vi "标样核查配置.vi"() -> (2 "确认输出":bool)   [LabVIEW 2022 SP3, in "斯坦道多参数.lvlib"]
panel:
  in  "余氯标样值":dbl caption="余氯"
  in  "余氯启用":bool
  in  "水中油标样值":dbl caption="水中油"
  in  "水中油启用":bool
  in  "悬浮物标样值":dbl caption="悬浮物"
  in  "悬浮物启用":bool
  in  "氨氮标样值":dbl caption="氨氮"
  in  "COD标样值":dbl caption="COD"
  in  "氨氮启用":bool
  in  "COD启用":bool
  in  "氯化物标样值":dbl caption="氯化物"
  in  "氯化物启用":bool
  in  "ORP标样值":dbl caption="ORP"
  in  "ORP启用":bool
  in  "藻密度标样值":dbl caption="藻密度"
  in  "叶绿素a标样值":dbl caption="叶绿素a"
  in  "藻密度启用":bool
  in  "叶绿素a启用":bool
  in  "保存组数":dbl=1.0
  in  "浊度启用":bool
  in  "电导率启用":bool
  in  "溶解氧启用":bool
  in  "pH启用":bool
  in  "浊度标样值":dbl caption="浊度"
  in  "电导率标样值":dbl caption="电导率"
  in  "溶解氧标样值":dbl caption="溶解氧"
  in  "pH标样值":dbl caption="pH"
  in  "取消":bool
  in  "确定":bool
  in  "数据保存间隔":dbl=1.0
  # "请输入数据保存间隔"
  # "保存组数"
  # "min"
  # "组"
  # "请选择启动项"
  # "请输入各参数标样值"
  # "mg/L"
  # "μS/cm"
  # "NTU"
  # "μg/L"
  # "cells/mL"
  # "mg/L"
  # "mg/L"
  # "mg/L"
  # "mg/L"
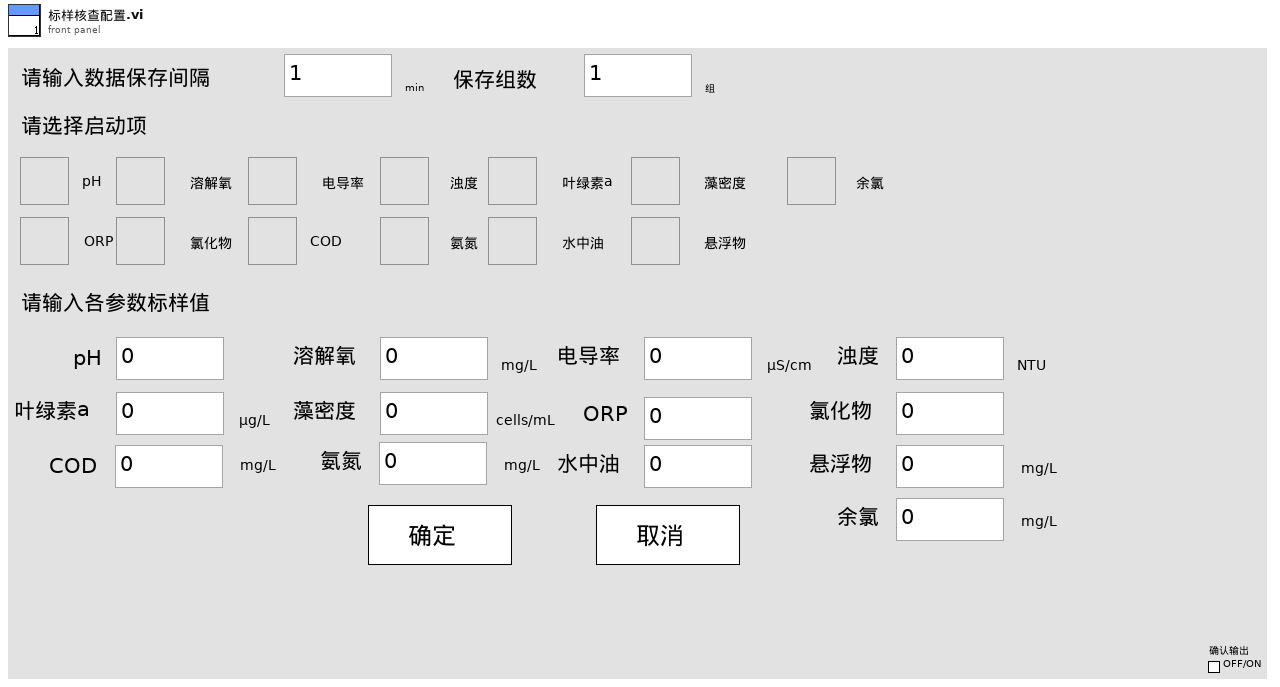
[diagram p1: front panel]
types:
  T1 = cluster{"数据保存间隔":dbl, "保存组数":dbl, "水温标样值":dbl, "pH标样值":dbl, "溶解氧标样值":dbl, "电导率标样值":dbl, "浊度标样值":dbl, "悬浮物标样值":dbl, "叶绿素a标样值":dbl, "藻密度标样值":dbl, "ORP标样值":dbl, "氯化物标样值":dbl, "COD标样值":dbl, "氨氮标样值":dbl, "水中油标样值":dbl, "余氯标样值":dbl, "pH启用":bool, "溶解氧启用":bool, "电导率启用":bool, "浊度启用":bool, "悬浮物启用":bool, "叶绿素a启用":bool, "藻密度启用":bool, "ORP启用":bool, "氯化物启用":bool, "COD启用":bool, "氨氮启用":bool, "水中油启用":bool, "余氯启用":bool}
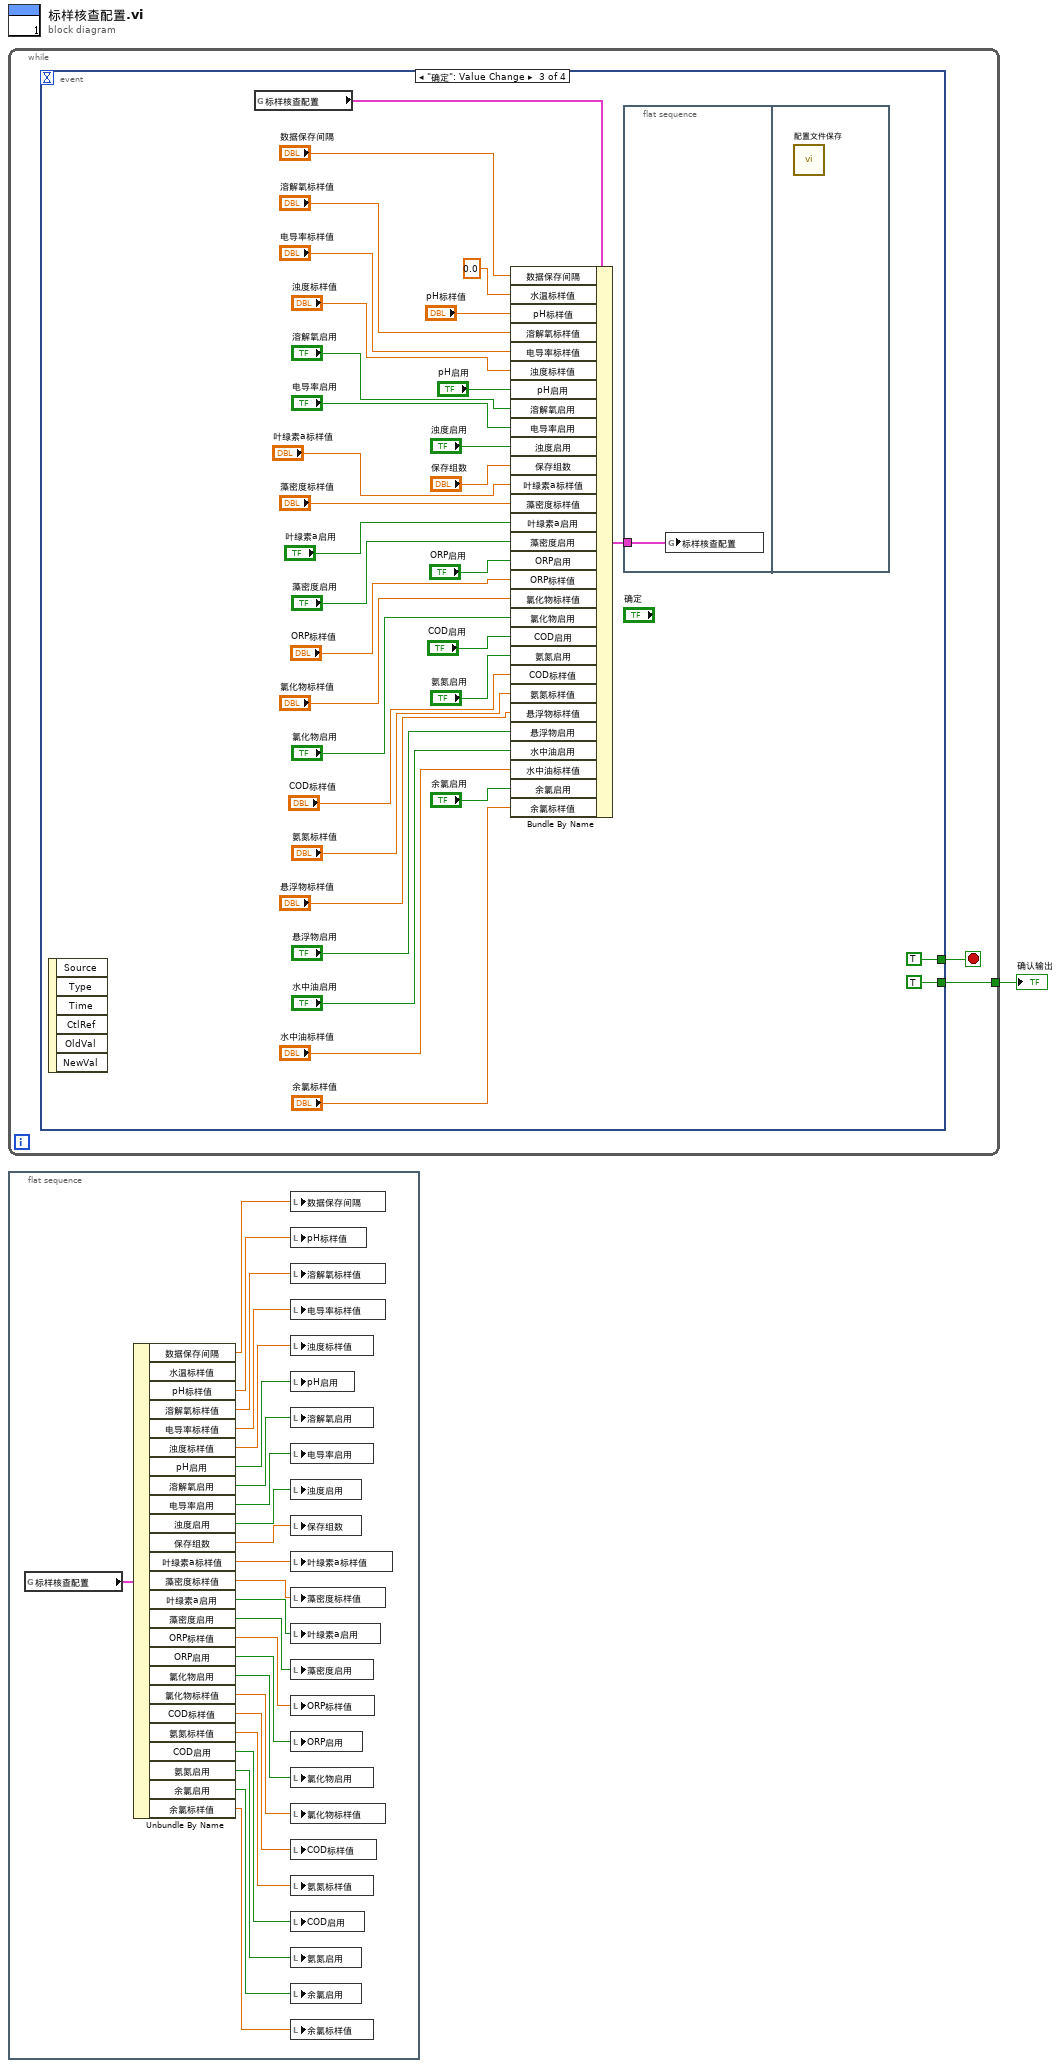
[diagram p0: block diagram]
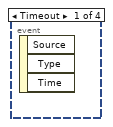
[diagram p2: hidden frame]
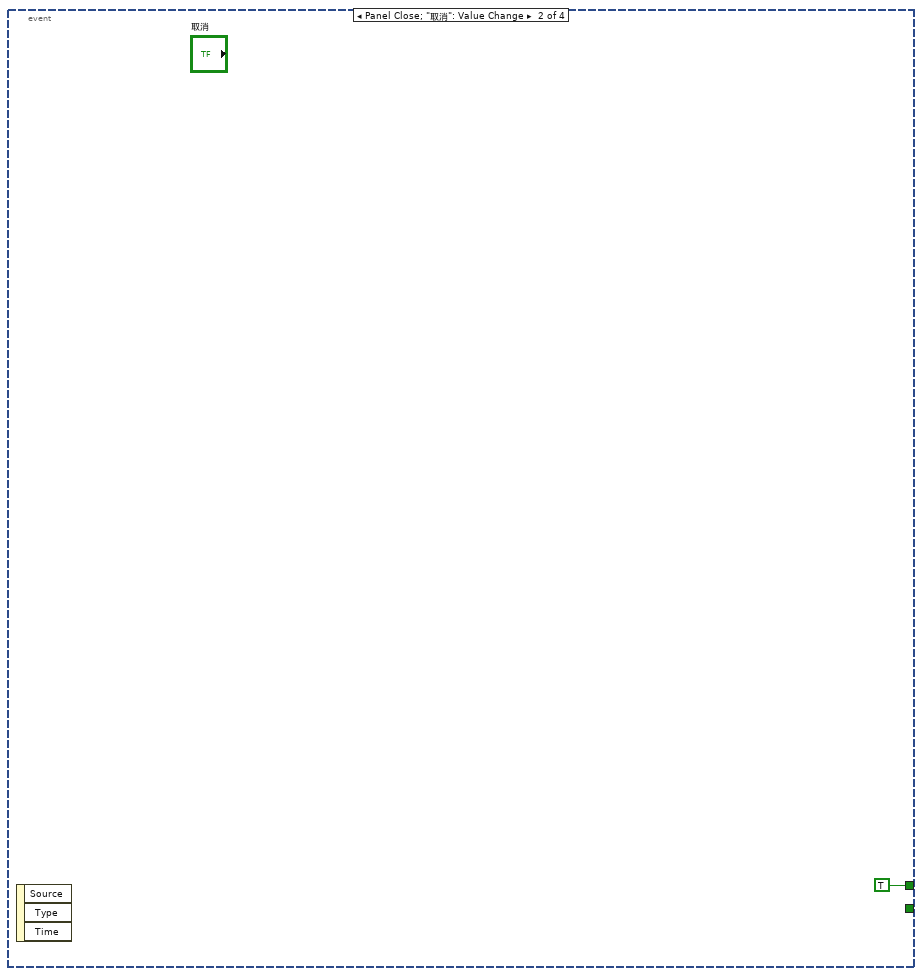
[diagram p3: hidden frame]
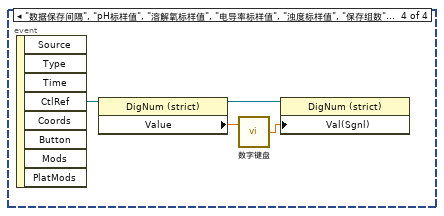
[diagram p4: hidden frame]
diagram:
  n1 = while {
    tunnel: [w2] -> w1
    stop <- w3 stop-if-true
    n2 = event shown="[2] \"确定\": Value Change" {
      selector: _ -> [_ _ _ _]
      dyn-events: _ -> [_ _ _ _]
      timeout: _ -> [_ _ _ _]
      tunnel: [_ TRUE TRUE _] -> w3
      tunnel: [_ _ TRUE _] -> w2
      event Timeout {
        n3 = event-data() -> ()  [unwired: 1 in, 3 out]
      }
      event Panel Close; "取消": Value Change {
        n4 = event-data() -> ()  [unwired: 1 in, 3 out]
      }
      event "确定": Value Change {
        n5 = event-data() -> ()  [unwired: 1 in, 6 out]
        n6 = global read "断电保存变量.vi" "标样核查配置"() -> (w36:T1)
        n7 = Bundle By Name(cluster=w36, "数据保存间隔"="数据保存间隔", "水温标样值"=0.0, "pH标样值"="pH标样值", "溶解氧标样值"="溶解氧标样值", "电导率标样值"="电导率标样值", "浊度标样值"="浊度标样值", "pH启用"="pH启用", "溶解氧启用"="溶解氧启用", "电导率启用"="电导率启用", "浊度启用"="浊度启用", "保存组数"="保存组数", "叶绿素a标样值"="叶绿素a标样值", "藻密度标样值"="藻密度标样值", "叶绿素a启用"="叶绿素a启用", "藻密度启用"="藻密度启用", "ORP启用"="ORP启用", "ORP标样值"="ORP标样值", "氯化物标样值"="氯化物标样值", "氯化物启用"="氯化物启用", "COD启用"="COD启用", "氨氮启用"="氨氮启用", "COD标样值"="COD标样值", "氨氮标样值"="氨氮标样值", "悬浮物标样值"="悬浮物标样值", "悬浮物启用"="悬浮物启用", "水中油启用"="水中油启用", "水中油标样值"="水中油标样值", "余氯启用"="余氯启用", "余氯标样值"="余氯标样值") -> (w35:T1)
        n8 = flat-sequence {
          tunnel: w35 -> [w38]
          frame #0 {
            n9 = global write "断电保存变量.vi" "标样核查配置"(w38) -> ()
          }
          frame #1 {
            n10 = call "配置文件保存.vi"() -> ()  [unwired: 12 in]
          }
        }
      }
      event "数据保存间隔", "pH标样值", "溶解氧标样值", "电导率标样值", "浊度标样值", "保存组数", "ORP标样值", "氯化物标样值": Mouse Down {
        n11 = event-data() -> ("CtlRef"=w42:refnum<vi>)  [unwired: 1 in, 7 out]
        n12 = property class="DigNum (strict)"(reference=w42) -> (reference out=w39:refnum<vi>, "Value"=w41:dbl)  [unwired: 1 in, 1 out]
        n13 = call "数字键盘.vi"("OldNumber"=w41) -> ("NewNumber"=w40:dbl)  [unwired: 1 in]
        n14 = property class="DigNum (strict)"(reference=w39, "Val(Sgnl)"=w40) -> ()  [unwired: 1 in, 2 out]
      }
    }
  }
  "确认输出" <- w1
  n15 = flat-sequence {
    frame #0 {
      n16 = global read "断电保存变量.vi" "标样核查配置"() -> (w67:T1)
      n17 = Unbundle By Name(w67) -> ("数据保存间隔"=w66:dbl, "pH标样值"=w62:dbl, "溶解氧标样值"=w63:dbl, "电导率标样值"=w64:dbl, "浊度标样值"=w65:dbl, "pH启用"=w61:bool, "溶解氧启用"=w60:bool, "电导率启用"=w59:bool, "浊度启用"=w58:bool, "保存组数"=w57:dbl, "叶绿素a标样值"=w56:dbl, "藻密度标样值"=w55:dbl, "叶绿素a启用"=w54:bool, "藻密度启用"=w53:bool, "ORP标样值"=w52:dbl, "ORP启用"=w51:bool, "氯化物启用"=w49:bool, "氯化物标样值"=w50:dbl, "COD标样值"=w48:dbl, "氨氮标样值"=w45:dbl, "COD启用"=w47:bool, "氨氮启用"=w46:bool, "余氯启用"=w44:bool, "余氯标样值"=w43:dbl)  [unwired: 1 out]
      n18 = local write "数据保存间隔"(w66) -> ()
      n19 = local write "pH标样值"(w62) -> ()
      n20 = local write "溶解氧标样值"(w63) -> ()
      n21 = local write "电导率标样值"(w64) -> ()
      n22 = local write "浊度标样值"(w65) -> ()
      n23 = local write "pH启用"(w61) -> ()
      n24 = local write "溶解氧启用"(w60) -> ()
      n25 = local write "电导率启用"(w59) -> ()
      n26 = local write "浊度启用"(w58) -> ()
      n27 = local write "保存组数"(w57) -> ()
      n28 = local write "叶绿素a标样值"(w56) -> ()
      n29 = local write "藻密度标样值"(w55) -> ()
      n30 = local write "叶绿素a启用"(w54) -> ()
      n31 = local write "藻密度启用"(w53) -> ()
      n32 = local write "ORP标样值"(w52) -> ()
      n33 = local write "ORP启用"(w51) -> ()
      n34 = local write "氯化物启用"(w49) -> ()
      n35 = local write "氯化物标样值"(w50) -> ()
      n36 = local write "COD标样值"(w48) -> ()
      n37 = local write "氨氮标样值"(w45) -> ()
      n38 = local write "COD启用"(w47) -> ()
      n39 = local write "氨氮启用"(w46) -> ()
      n40 = local write "余氯启用"(w44) -> ()
      n41 = local write "余氯标样值"(w43) -> ()
    }
  }
